vi "svx_Orbit Attribute_NOLIB.vi"(0 "attribute":variant) -> (14 "probe angle X":dbl, 15 "probe angle Y":dbl, 16 "rotating direction":u16, 17 "samples/rev":dbl, 18 "pair":string, 19 "order":string)   [LabVIEW 2017]
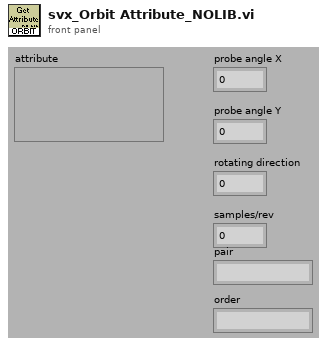
[diagram p1: front panel]
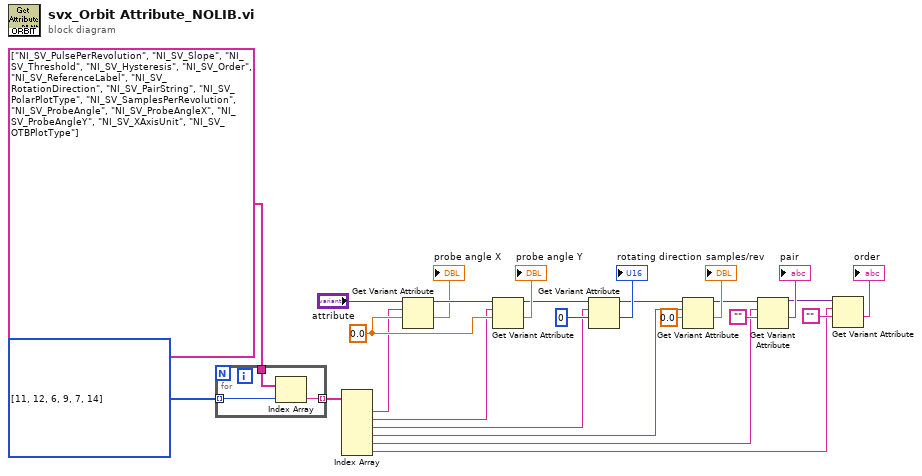
[diagram p0: block diagram]
diagram:
  w8 = u16[] [11, 12, 6, 9, 7, 14] items=["Pulse / Revolution", "Slope", "Threshold", "Hysteresis", "Order", "Reference Label", "Rotation Direction", "Pair String", "Polar Plot Type", "Sample Per Revolution", "Probe Angle", "Probe Angle X", "Probe Angle Y", "X Axis Unit", "OTB Plot Type"]
  w10 = 0.0 ("pair")
  n1 = for {
    tunnel: string[] ["NI_SV_PulsePerRevolution", "NI_SV_Slope", "NI_SV_Threshold", "NI_SV_Hysteresis", "NI_SV_Order", "NI_SV_ReferenceLabel", "NI_SV_RotationDirection", "NI_SV_PairString", "NI_SV_PolarPlotType", "NI_SV_SamplesPerRevolution", "NI_SV_ProbeAngle", "NI_SV_ProbeAngleX", "NI_SV_ProbeAngleY", "NI_SV_XAxisUnit", "NI_SV_OTBPlotType"] -> [w29]
    tunnel: w8 -> [w28] mode=indexing
    tunnel: [w27] -> w7 mode=indexing
    n2 = Index Array(array=w29, index=w28) -> (element=w27:string)
  }
  n3 = Index Array(array=w7) -> (element #1=w6:string, element #2=w5:string, element #3=w4:string, element #4=w3:string, element #5=w2:string, element #6=w1:string)  [unwired: 6 in]
  n4 = Get Variant Attribute(Variant="attribute", name=w6, default value (empty Variant)=w10) -> (duplicate Variant=w26:variant, value=→"probe angle X":dbl)  [unwired: 1 in, 2 out]
  n5 = Get Variant Attribute(Variant=w26, name=w5, default value (empty Variant)=w10) -> (duplicate Variant=w22:variant, value=→"probe angle Y":dbl)  [unwired: 1 in, 2 out]
  n6 = Get Variant Attribute(Variant=w22, name=w4, default value (empty Variant)=u16 0 ("direction")) -> (duplicate Variant=w19:variant, value=→"rotating direction":u16)  [unwired: 1 in, 2 out]
  n7 = Get Variant Attribute(Variant=w19, name=w3, default value (empty Variant)=0.0 ("pair")) -> (duplicate Variant=w18:variant, value=→"samples/rev":dbl)  [unwired: 1 in, 2 out]
  n8 = Get Variant Attribute(Variant=w18, name=w2, default value (empty Variant)="") -> (duplicate Variant=w14:variant, value=→"pair":string)  [unwired: 1 in, 2 out]
  n9 = Get Variant Attribute(Variant=w14, name=w1, default value (empty Variant)="") -> (value=→"order":string)  [unwired: 1 in, 3 out]
